vi "Error Prefix.vi"(10 "VI Ref":refnum<vi>) -> (2 "Prefix":string)   [LabVIEW 2025, in "jettl.lvlib" / "Error.lvlib"]
uses:
  Error.lvlib
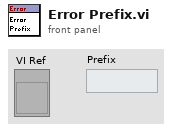
[diagram p1: front panel]
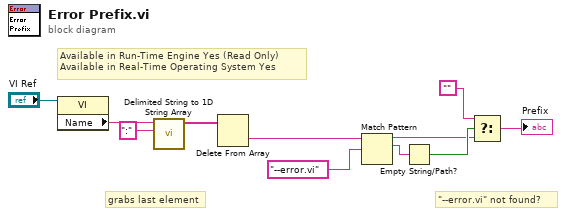
[diagram p0: block diagram]
diagram:
  # "grabs last element"
  # "Available in Run-Time Engine Yes (Read Only) \nAvailable in Real-Time Operating System Yes"
  # "\"--error.vi\" not found?"
  n1 = property class="VI"(reference="VI Ref") -> ("Name"=w2:string)  [unwired: 1 in, 2 out]
  n2 = call <vilib>:"Delimited String to 1D String Array.vi"("delimiter"=":", "delimited string"=w2) -> ("string array"=w9:string[])  [unwired: 9 in]
  n3 = Delete From Array "Delete From Array"(array=w9) -> (deleted portion=w8:string)  [unwired: 2 in, 1 out]
  n4 = Match Pattern(string=w8, regular expression="--error.vi") -> (before substring=w5:string, match substring=w11:string)  [unwired: 1 in, 2 out]
  n5 = Empty String/Path?(string/path=w11) -> (empty?=w6:bool)
  n6 = Select(t="", s=w6, f=w5) -> (s? t:f=→"Prefix":string)
